vi "PerformCalibration.vi"(0 "MFCS_EZ":T3, 1 "Total Flow Setpoint":dbl, 2 "Ctr Water Valve":u16(ring) items=["A1", "A2", "A3", "A4", "B1", "B2", "B3", "B4", "B5", "B6", "B7", "B8", "A5", "A6", "A7", "A8"], 3 "Calibration Mode":T2(ring), 5 "Calibration Refs":T1, 7 "Manual Default Set Pressures":dbl[](array[numeric]), 12 "Total Odor Flow":dbl, 13 "Water Mix Valve":u16(ring) items=["A1", "A2", "A3", "A4", "B1", "B2", "B3", "B4", "B5", "B6", "B7", "B8", "A5", "A6", "A7", "A8", ""]) -> (4 "Ctr Pressure":dbl, 6 "Set Pressures":dbl[][](array[numeric]), 15 "Aborted?":bool)   [LabVIEW 2016]
uses:
  <userlib>/Fluigent/Fluigent MFCS/FluigentMFCS_Full.llb/_EZmfcsRefNum.ctl
  <userlib>/Fluigent/Fluigent MFCS/FluigentMFCS_Full.llb/_EZmfcsEnum.ctl
  <userlib>/Fluigent/Fluigent MFCS/FluigentMFCS_Full.llb/MFCS_EZ Write Channel Pressure.vi
  Globals/PressuresGlobal.vi
  <vilib>/Utility/miscctls.llb/LVStringsAndValuesArrayTypeDef.ctl
panel:
  out "odor starting pressure":dbl
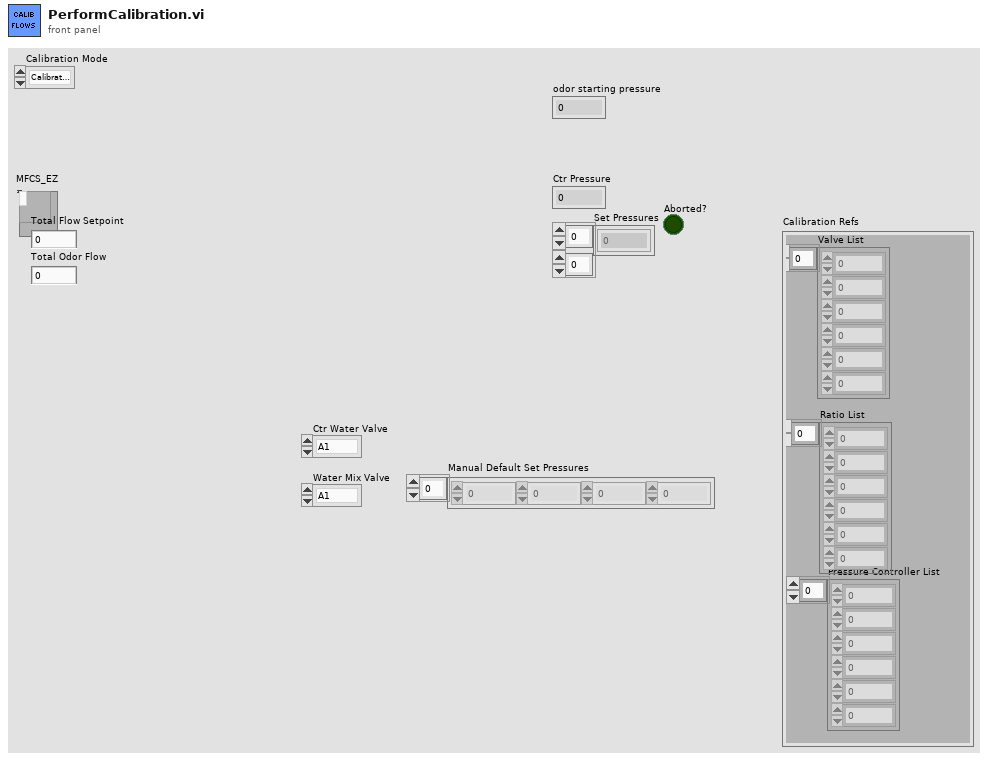
[diagram p1: front panel]
types:
  T1 = cluster{"Pressure Controller List":u8[], "Ratio List":dbl[], "Valve List":u16[]}
  T2 = enum16{"Calibrate All", "Control Only", "Odors Only"}
  T3 = typedef "_EZmfcsRefNum.ctl" = refnum<k1>
  T4 = typedef "LVStringsAndValuesArrayTypeDef.ctl" = cluster{"String":string, "Value":ext}[]
  T5 = enum16{"Release", "Create", "Send", "Wait", "Cancel"}
  T6 = cluster{enum16{"A", "B", "C"}[], enum16{"1", "2", "3", "4", "5", "6", "7", "8"}[], bool[]}
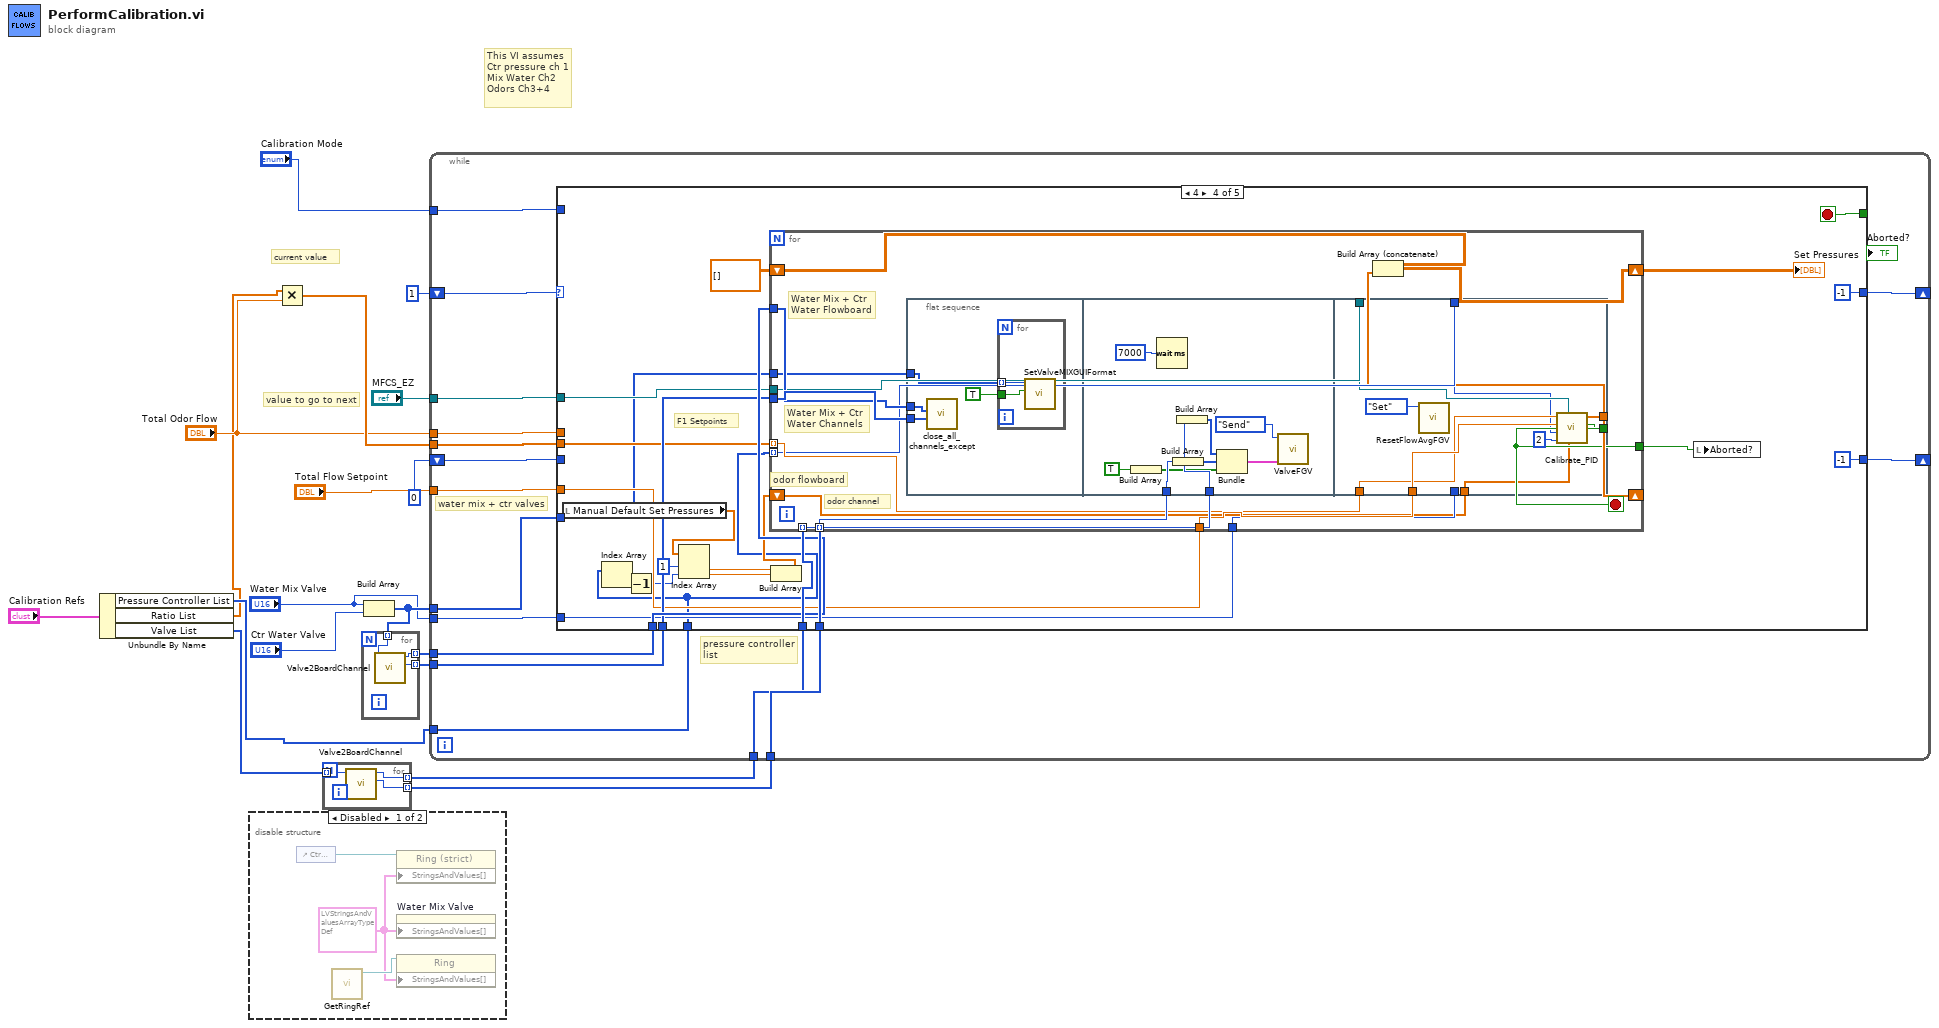
[diagram p0: block diagram]
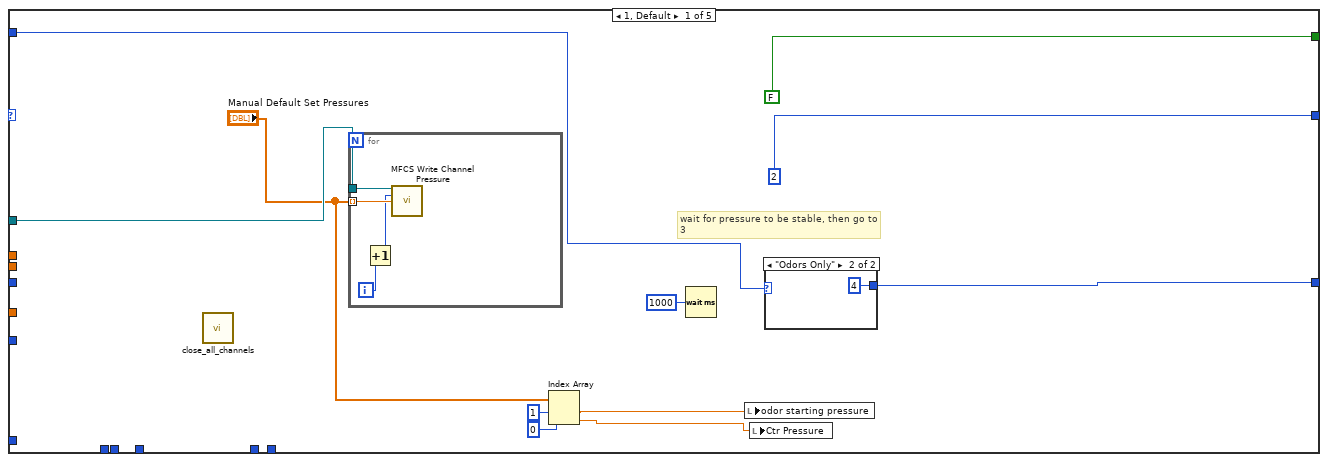
[diagram p3: hidden frame]
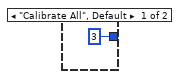
[diagram p4: hidden frame]
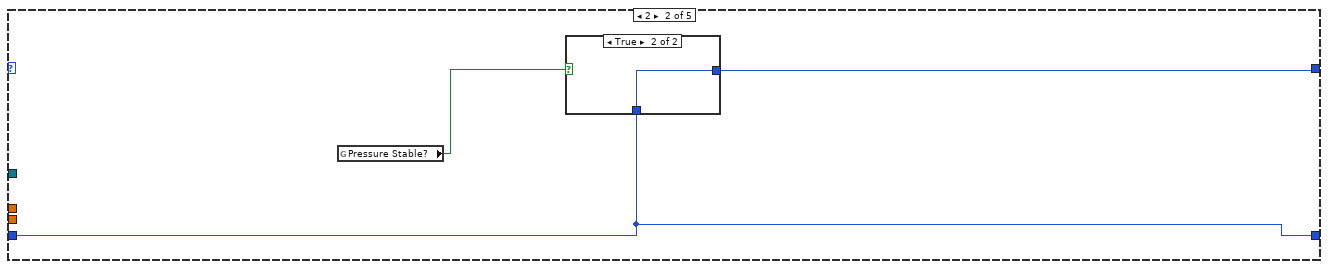
[diagram p5: hidden frame]
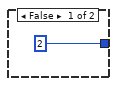
[diagram p6: hidden frame]
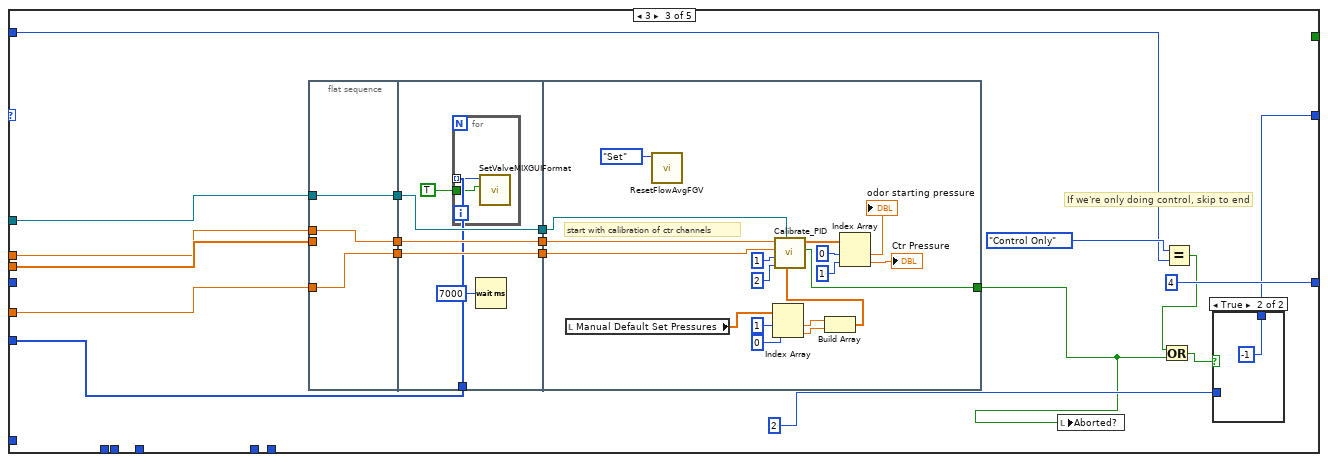
[diagram p7: hidden frame]
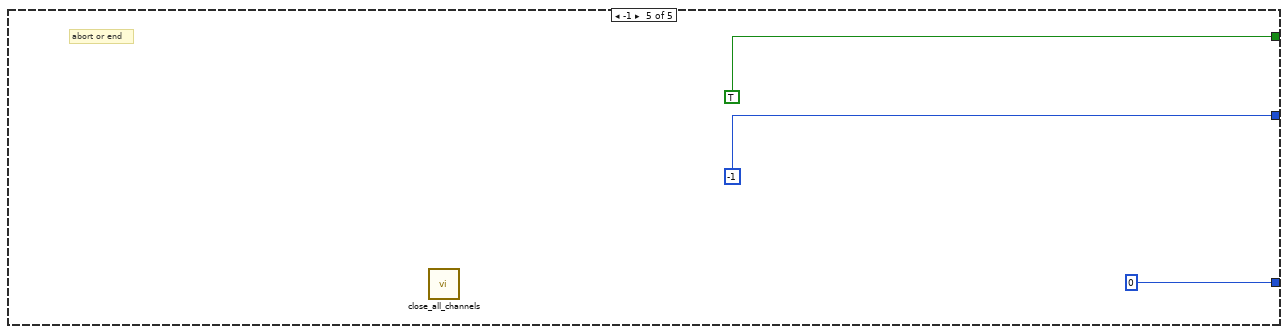
[diagram p9: hidden frame]
diagram:
  # "This VI assumes \nCtr pressure ch 1\nMix Water Ch2\nOdors Ch3+4"
  # "current value"
  # "value to go to next"
  n1 = Unbundle By Name("Calibration Refs") -> ("Pressure Controller List"=w3:u8[], "Ratio List"=w1:dbl[], "Valve List"=w2:u16[])
  n2 = disable-structure shown="Disabled" {
    frame Disabled {
      w19 = T4 [{"String"="A1", "Value"=0.0}, {"String"="A2", "Value"=1.0}, {"String"="A3", "Value"=2.0}, {"String"="A4", "Value"=3.0}, {"String"="B1", "Value"=4.0}, {"String"="B2", "Value"=5.0}, {"String"="B3", "Value"=6.0}, {"String"="B4", "Value"=7.0}, {"String"="B5", "Value"=8.0}, {"String"="B6", "Value"=9.0}, {"String"="B7", "Value"=10.0}, {"String"="B8", "Value"=11.0}, {"String"="A5", "Value"=12.0}] ("Master Valves")
      n3 = control-ref of="Ctr Water Valve"() -> (w20:refnum<vi>)
      n4 = call "GetRingRef.vi"() -> ("Ring Reference"=w21:refnum<vi>, "Array Reference"=w22:refnum<vi>)  [unwired: 9 in, 1 out]
      n5 = property on="Property Node" class="Ring (strict)"(reference=w20, "StringsAndValues[]"=w19) -> ()  [unwired: 1 in, 2 out]
      n6 = property on="Water Mix Valve" class="Ring (strict)"("StringsAndValues[]"=w19) -> ()  [unwired: 2 in, 2 out]
      n7 = property class="Ring"(reference=w21, "StringsAndValues[]"=w19) -> ()  [unwired: 1 in, 2 out]
    }
    frame Enabled {
    }
  }
  n8 = Multiply(x=w1, y="Total Odor Flow") -> (x*y=w8:dbl[])
  n9 = for {
    tunnel: w2 -> [w25] mode=indexing
    tunnel: [w24] -> w12 mode=indexing
    tunnel: [w23] -> w13 mode=indexing
    n10 = call "Valve2BoardChannel.vi"("ValveID"=w25) -> ("Channel"=w23:enum16{"1", "2", "3", "4", "5", "6", "7", "8"}, "Flowboard"=w24:enum16{"A", "B", "C"})  [unwired: 9 in]
  }
  n11 = Build Array("Water Mix Valve", "Ctr Water Valve") -> (w11:u16[])
  n12 = for {
    tunnel: w11 -> [w28] mode=indexing
    tunnel: [w27] -> w10 mode=indexing
    tunnel: [w26] -> w9 mode=indexing
    n13 = call "Valve2BoardChannel.vi"("ValveID"=w28) -> ("Channel"=w26:enum16{"1", "2", "3", "4", "5", "6", "7", "8"}, "Flowboard"=w27:enum16{"A", "B", "C"})  [unwired: 9 in]
  }
  n14 = while {
    tunnel: "MFCS_EZ" -> [w45]
    tunnel: "Total Flow Setpoint" -> [w44]
    shift-right: [w41] -> _
    shift-left: 1 -> [w43]
    tunnel: w11 -> [w40]
    shift-right: [w39] -> _
    shift-left: 0 -> [w38]
    tunnel: w3 -> [w29]
    tunnel: w13 -> [w37]
    tunnel: w12 -> [w36]
    tunnel: w10 -> [w35]
    tunnel: w9 -> [w34]
    tunnel: w8 -> [w33]
    tunnel: "Water Mix Valve" -> [w31]
    tunnel: "Total Odor Flow" -> [w32]
    tunnel: "Calibration Mode" -> [w30]
    stop <- w42 stop-if-true
    # "pressure controller \nlist"
    # "water mix + ctr valves"
    n15 = case shown="4" w43 {
      tunnel: w45 -> [w54 _ w86 w134 _]
      tunnel: w33 -> [_ _ w85 w133 _]
      tunnel: w44 -> [_ _ w84 w135 _]
      tunnel: [FALSE _ _ _ TRUE] -> w42
      tunnel: [2 w64 w74 -1 -1] -> w41
      tunnel: w40 -> [_ _ w68 w125 _]
      tunnel: [w53 w63 4 -1 0] -> w39
      tunnel: w38 -> [_ w63 _ _ _]
      tunnel: w29 -> [_ _ _ w122 _]
      tunnel: w37 -> [_ _ _ w139 _]
      tunnel: w36 -> [_ _ _ w138 _]
      tunnel: w35 -> [_ _ _ w137 _]
      tunnel: w34 -> [_ _ _ w136 _]
      tunnel: w31 -> [_ _ _ w132 _]
      tunnel: w32 -> [_ _ w77 _ _]
      tunnel: w30 -> [w51 _ w71 _ _]
      frame 1, Default {
        # "wait for pressure to be stable, then go to\n3"
        n16 = call "close_all_channels.vi"() -> ()  [unwired: 12 in]
        n17 = for {
          tunnel: "Manual Default Set Pressures" -> [w62] mode=indexing
          tunnel: w54 -> [w60]
          i -> [w61]
          n18 = Increment(x=w61) -> (x+1=w59:i32)
          n19 = call-poly <userlib>:"MFCS Write Channel Pressure.vi"("MFCS_EZ"=w60, "Channel Number (default=1)"=w59, "Pressure (mBar)"=w62) -> ()  [unwired: 11 in, 2 out]
        }
        n20 = Index Array(array="Manual Default Set Pressures", index #1=1 ("index"), index #2=0 ("index")) -> (element #1=w47:dbl, element #2=w46:dbl)
        n21 = Wait (ms)(milliseconds to wait=u32 1000) -> ()  [unwired: 1 out]
        n22 = local write "odor starting pressure"(w47) -> ()
        n23 = local write "Ctr Pressure"(w46) -> ()
        n24 = case shown="\"Odors Only\"" w51 {
          tunnel: [3 4] -> w53
          frame "Calibrate All", Default {
          }
          frame "Odors Only" {
          }
        }
      }
      frame 2 {
        n25 = global read "PressuresGlobal.vi" "Pressure Stable?"() -> (w65:bool)
        n26 = case shown="True" w65 {
          tunnel: [2 w67] -> w64
          tunnel: w63 -> [_ w67]
          frame False {
          }
          frame True {
          }
        }
      }
      frame 3 {
        # "If we're only doing control, skip to end"
        n27 = flat-sequence {
          tunnel: w84 -> [w90]
          tunnel: w85 -> [_]
          tunnel: w86 -> [w91]
          tunnel: [w91] -> w83
          tunnel: [w90] -> w80
          tunnel: w77 -> [w89]
          tunnel: [w89] -> w76
          tunnel: w83 -> [w97]
          tunnel: [w97] -> w82
          tunnel: [w96] -> w81
          tunnel: w80 -> [w95]
          tunnel: [w95] -> w79
          tunnel: w68 -> [w93]
          tunnel: w76 -> [w96]
          tunnel: w82 -> [w117]
          tunnel: w81 -> [w116]
          tunnel: w79 -> [w115]
          tunnel: [w101] -> w69
          frame #0 {
          }
          frame #1 {
            n28 = for {
              tunnel: TRUE ("State") -> [w99]
              tunnel: w93 -> [w98] mode=indexing
              n29 = call "SetValveMIXGUIFormat.vi"("State"=w99, "ValveID"=w98) -> ()  [unwired: 10 in]
            }
            n30 = Wait (ms)(milliseconds to wait=u32 7000) -> ()  [unwired: 1 out]
          }
          frame #2 {
            # "start with calibration of ctr channels"
            n31 = local read "Manual Default Set Pressures"() -> (w108:dbl[])
            n32 = call "ResetFlowAvgFGV.vi"("Action"=enum16{"Create", "Set", "Wait"}."Set") -> ()  [unwired: 10 in, 1 out]
            n33 = Index Array(array=w108, index #1=1 ("index"), index #2=0 ("index")) -> (element #1=w104:dbl, element #2=w105:dbl)
            n34 = Build Array(w104, w105) -> (w103:dbl[])
            n35 = call "Calibrate_PID.vi"("Starting Pressure"=w103, "MFCS_EZ"=w117, "Water Mix Pressure Channel"=i16 2, "Odor Mix Pressure Channel"=i16 1, "Ftot Setpoint"=w115, "F1 Setpoint"=w116) -> ("Aborted?"=w101:bool, "Set Pressure Out"=w112:dbl[])  [unwired: 4 in]
            n36 = Index Array(array=w112, index #1=0 ("index"), index #2=1 ("index")) -> (element #1=→"odor starting pressure":dbl, element #2=→"Ctr Pressure":dbl)
          }
        }
        n37 = local write "Aborted?"(w69) -> ()
        n38 = Equal?(x=T2."Control Only" ("Calibration Mode"), y=w71) -> (x = y?=w70:bool)
        n39 = Or(x=w70, y=w69) -> (x .or. y?=w73:bool)
        n40 = case shown="True" w73 {
          tunnel: 2 -> [w87 _]
          tunnel: [w87 -1] -> w74
          frame False {
          }
          frame True {
          }
        }
      }
      frame 4 {
        # "F1 Setpoints"
        n41 = local read "Manual Default Set Pressures"() -> (w124:dbl[])
        n42 = Index Array(array=w122) -> (element=w121:u8)  [unwired: 1 in]
        n43 = Decrement(x=w121) -> (x-1=w120:u8)
        n44 = Index Array(array=w124, index #1=1 ("index"), index #2=w120) -> (element #1=w118:dbl, element #2=w119:dbl)
        n45 = Build Array(w118, w119) -> (w127:dbl[])
        n46 = for {
          tunnel: w122 -> [w147] mode=indexing
          tunnel: w139 -> [w151] mode=indexing
          tunnel: w138 -> [w152] mode=indexing
          tunnel: w137 -> [w153]
          tunnel: w136 -> [w154]
          tunnel: w135 -> [w150]
          tunnel: w134 -> [w149]
          tunnel: w133 -> [w148] mode=indexing
          tunnel: w132 -> [w146]
          shift-right: [w145] -> w130
          shift-left: dbl[][] [] -> [w144]
          shift-right: [w143] -> _
          shift-left: w127 -> [w142]
          tunnel: [w141] -> w126
          tunnel: w125 -> [w140]
          stop <- w141 stop-if-true
          # "odor channel"
          # "odor flowboard"
          # "Water Mix + Ctr \nWater Channels"
          # "Water Mix + Ctr \nWater Flowboard"
          n47 = flat-sequence {
            tunnel: w154 -> [w158]
            tunnel: w153 -> [w157]
            tunnel: w140 -> [w155]
            tunnel: w152 -> [w166]
            tunnel: w151 -> [w167]
            tunnel: w150 -> [w178]
            tunnel: w149 -> [w177]
            tunnel: w148 -> [w176]
            tunnel: [w175] -> w141
            tunnel: [w174] -> w143
            tunnel: w147 -> [w173]
            tunnel: w146 -> [_]
            tunnel: w142 -> [w171]
            frame #0 {
              n48 = call "close_all_channels_except.vi"("Channel"=w158, "Flowboard"=w157) -> ()  [unwired: 10 in]
              n49 = for {
                tunnel: TRUE ("State") -> [w160]
                tunnel: w155 -> [w159] mode=indexing
                n50 = call "SetValveMIXGUIFormat.vi"("State"=w160, "ValveID"=w159) -> ()  [unwired: 10 in]
              }
            }
            frame #1 {
              n51 = Build Array(TRUE ("State")) -> (w163:bool[])
              n52 = Wait (ms)(milliseconds to wait=u32 7000) -> ()  [unwired: 1 out]
              n53 = Build Array(w167) -> (w164:enum16{"1", "2", "3", "4", "5", "6", "7", "8"}[])
              n54 = Build Array(w166) -> (w165:enum16{"A", "B", "C"}[])
              n55 = Bundle(w165, w164, w163) -> (w162:T6)  [unwired: 1 in]
              n56 = call "ValveFGV.vi"("Valve Data"=w162, "Action"=T5."Send") -> ()  [unwired: 6 in, 4 out]
            }
            frame #2 {
              n57 = call "ResetFlowAvgFGV.vi"("Action"=enum16{"Create", "Set", "Wait"}."Set") -> ()  [unwired: 10 in, 1 out]
              n58 = call "Calibrate_PID.vi"("Starting Pressure"=w171, "MFCS_EZ"=w177, "Water Mix Pressure Channel"=i16 2, "Odor Mix Pressure Channel"=w173, "Ftot Setpoint"=w178, "F1 Setpoint"=w176) -> ("Aborted?"=w175:bool, "Set Pressure Out"=w174:dbl[])  [unwired: 4 in]
            }
          }
          n59 = Build Array (concatenate)(w144, w143) -> (w145:dbl[][])
        }
        "Set Pressures" <- w130
        n60 = local write "Aborted?"(w126) -> ()
      }
      frame -1 {
        # "abort or end"
        n61 = call "close_all_channels.vi"() -> ()  [unwired: 12 in]
      }
    }
  }
